vi "BuildStrings_Return.vi"(4 "seconds to wait":dbl format="%#_13g", 7 "Input String":string, 8 "New String":string="\n\n", 9 "error in (no error)":errorcluster, 11 "reference":refnum<vi>) -> (0 "error out":errorcluster, 1 "concatenated string":string, 3 "reference out":refnum<vi>)   [LabVIEW 2018]
panel:
  in  "ClearErrors(t)":bool=TRUE
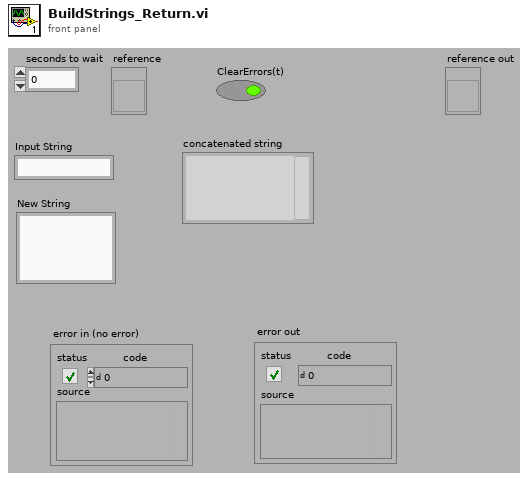
[diagram p1: front panel]
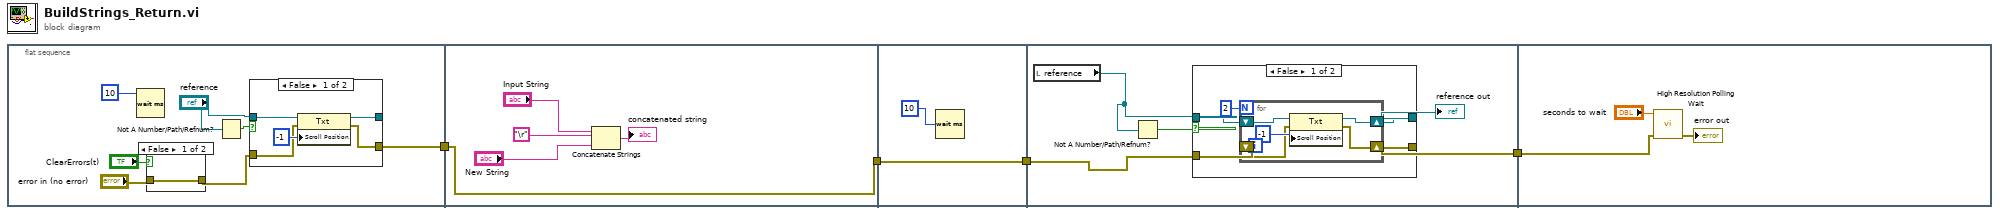
[diagram p0: block diagram]
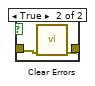
[diagram p2: hidden frame]
diagram:
  n1 = flat-sequence {
    tunnel: [w7] -> w3
    tunnel: [w22] -> w2
    tunnel: w3 -> [w22]
    tunnel: w2 -> [w28]
    tunnel: [w28] -> w1
    tunnel: w1 -> [w31]
    tunnel: [w29] -> w4
    tunnel: w4 -> [w47]
    frame #0 {
      n2 = Wait (ms)(milliseconds to wait=u32 10) -> ()  [unwired: 1 out]
      n3 = case shown="False" "ClearErrors(t)" {
        tunnel: "error in (no error)" -> [w12 w14]
        tunnel: [w12 w13] -> w6
        frame False {
        }
        frame True {
          n4 = call <vilib>:"Clear Errors.vi"("error in (no error)"=w14) -> ("error out"=w13:errorcluster)  [unwired: 5 in, 1 out]
        }
      }
      n5 = Not A Number/Path/Refnum?(number/path/refnum="reference") -> (NaN/Path/Refnum?=w11:bool)
      n6 = case shown="False" w11 {
        tunnel: "reference" -> [w19 w20]
        tunnel: w6 -> [w17 w21]
        tunnel: [w16 w21] -> w7
        tunnel: [w15 w20] -> _
        frame False {
          n7 = property class="Txt"(reference=w19, error in=w17, "Scroll Position"=-1) -> (reference out=w15:refnum<vi>, error out=w16:errorcluster)
        }
        frame True {
        }
      }
    }
    frame #1 {
      n8 = Concatenate Strings("Input String", "\r", "New String") -> (→"concatenated string":string)
    }
    frame #2 {
      n9 = Wait (ms)(milliseconds to wait=u32 10) -> ()  [unwired: 1 out]
    }
    frame #3 {
      n10 = local read "reference"() -> (w32:refnum<vi>)
      n11 = Not A Number/Path/Refnum?(number/path/refnum=w32) -> (NaN/Path/Refnum?=w33:bool)
      n12 = case shown="False" w33 {
        tunnel: w32 -> [w38 w44]
        tunnel: w31 -> [w37 w45]
        tunnel: [w36 w45] -> w29
        tunnel: [w35 w44] -> w30
        frame False {
          n13 = for {
            N: 2 -> [_]
            shift-right: [w39] -> w35
            shift-left: w38 -> [w43]
            shift-right: [w40] -> w36
            shift-left: w37 -> [w41]
            n14 = property class="Txt"(reference=w43, error in=w41, "Scroll Position"=-1) -> (reference out=w39:refnum<vi>, error out=w40:errorcluster)
          }
        }
        frame True {
        }
      }
      "reference out" <- w30
    }
    frame #4 {
      n15 = call <vilib>:"High Resolution Polling Wait.vi"("error in (no error)"=w47, "seconds to wait"="seconds to wait") -> ("error out"=→"error out":errorcluster)  [unwired: 9 in]
    }
  }
